vi "FindMostRecent.vi"(8 "error in":errorcluster, 10 "Filename Pattern":string="VRM2014", 11 "Folder Path In":path=path "C:/VRM/logfiles") -> (0 "error out":errorcluster, 3 "File Path for the Newest File":path)   [LabVIEW 2013]
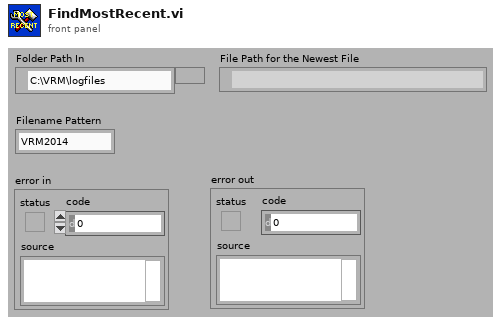
[diagram p1: front panel]
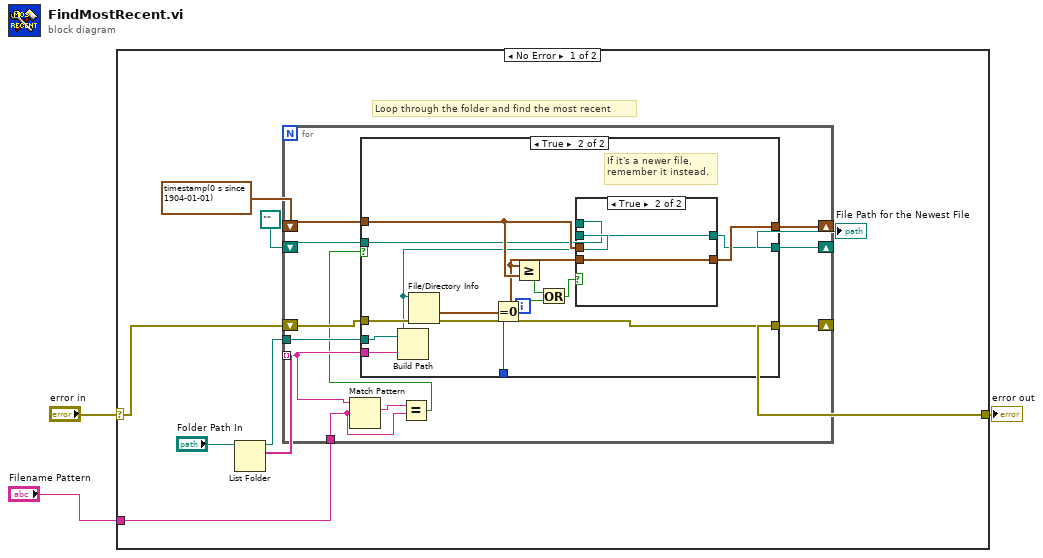
[diagram p0: block diagram]
diagram:
  n1 = case shown="No Error" "error in" {
    selector: "error in" -> [w8 w46]
    tunnel: [w12 w46] -> w3
    tunnel: "Filename Pattern" -> [w4 _]
    frame No Error {
      # "Loop through the folder and find the most recent"
      n2 = List Folder(path="Folder Path In") -> (path out=w6:path, filenames=w5:string[])  [unwired: 3 in, 2 out]
      n3 = for {
        shift-right: [w21] -> _
        shift-left: timestamp(0 s since 1904-01-01) ("last mod 2") -> [w22]
        shift-right: [w20] -> w11
        shift-left: path "" -> [w19]
        shift-right: [w18] -> w12
        shift-left: w8 -> [w24]
        tunnel: w5 -> [w16] mode=indexing
        tunnel: w6 -> [w17]
        tunnel: w4 -> [w13]
        i -> [w23]
        n4 = Match Pattern(string=w16, regular expression=w13) -> (match substring=w15:string)  [unwired: 1 in, 3 out]
        n5 = Equal?(x=w15, y=w13) -> (x = y?=w14:bool)
        n6 = case shown="True" w14 {
          tunnel: w24 -> [w25 w41]
          tunnel: w23 -> [_ w37]
          tunnel: w22 -> [w27 w36]
          tunnel: [w27 w35] -> w21
          tunnel: [w26 w32] -> w20
          tunnel: w19 -> [w26 w31]
          tunnel: [w25 w30] -> w18
          tunnel: w17 -> [_ w29]
          tunnel: w16 -> [_ w28]
          frame False {
          }
          frame True {
            # "If it's a newer file,\nremember it instead."
            n7 = Build Path(base path=w29, name or relative path=w28) -> (appended path=w33:path)
            n8 = File/Directory Info(path=w33, error in=w41) -> (last mod=w34:timestamp, error out=w30:errorcluster)  [unwired: 5 out]
            n9 = Equal To 0?(x=w37) -> (x = 0?=w38:bool)
            n10 = Greater Or Equal?(x=w34, y=w36) -> (x >= y?=w39:bool)
            n11 = Or(x=w39, y=w38) -> (x .or. y?=w40:bool)
            n12 = case shown="True" w40 {
              tunnel: w36 -> [w43 _]
              tunnel: [w43 w45] -> w35
              tunnel: w34 -> [_ w45]
              tunnel: w33 -> [_ w44]
              tunnel: [w42 w44] -> w32
              tunnel: w31 -> [w42 _]
              frame False {
              }
              frame True {
              }
            }
          }
        }
      }
      "File Path for the Newest File" <- w11
    }
    frame Error {
    }
  }
  "error out" <- w3
